vi "VDH-resetCalibrationValues.vi"(11 "VDH-VNA_data_handler in":refnum<class "VDH-VNA_data_handler.lvclass">) -> (3 "VDH-VNA_data_handler out":refnum<class "VDH-VNA_data_handler.lvclass">)   [LabVIEW 2020, in "VDH-VNA_data_handler.lvlib" / "VDH-VNA_data_handler.lvclass"]
uses:
  VDH-VNA_data_handler.lvclass
  VDH-Calibration_info.ctl
  VDH-Calibration_enum.ctl
  VDH-Calibration_factor.ctl
  VDH-calibration_status.ctl
  VDH-SOLT_calib_Status.ctl
  VDH-Calibration_prosess.ctl
  VDH-Calibration_temp_storage.ctl
  VDH-VNA_data_handler.lvclass/VDH-VNA_data_handler.ctl
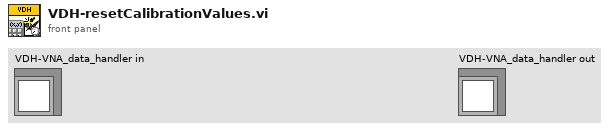
[diagram p1: front panel]
types:
  T1 = typedef "VDH-VNA_data_handler.lvlib/VDH-VNA_data_handler.lvclass/VDH-Calibration_temp_storage.ctl" = cluster{"S11":cdb[][], "Frequency":u64[]}
  T2 = typedef "VDH-VNA_data_handler.lvlib/VDH-VNA_data_handler.lvclass/VDH-calibration_status.ctl" = cluster{"Calib Status":T3, "Calibrated?":bool, "Permativity?":bool, "Progress":T4}
  T3 = typedef "VDH-VNA_data_handler.lvlib/VDH-VNA_data_handler.lvclass/VDH-SOLT_calib_Status.ctl" = cluster{"Short":bool, "Open":bool, "Load":bool, "Through":bool}
  T4 = typedef "VDH-VNA_data_handler.lvlib/VDH-VNA_data_handler.lvclass/VDH-Calibration_prosess.ctl" = cluster{"Progress":bool, "current":T5, "samples to get":u8}
  T5 = typedef "VDH-VNA_data_handler.lvlib/VDH-VNA_data_handler.lvclass/VDH-Calibration_enum.ctl" = enum16{"Non", "Short", "Open", "Load", "Through", "Permativity"}
  T6 = typedef "VDH-VNA_data_handler.lvlib/VDH-VNA_data_handler.lvclass/VDH-Calibration_factor.ctl" = cluster{"A":cdb[], "B":cdb[], "C":cdb[]}
  T7 = typedef "VDH-VNA_data_handler.lvlib/VDH-VNA_data_handler.lvclass/VDH-Calibration_info.ctl" = cluster{"map":map{T5, cdb[]}, "Frequency":u64[]}
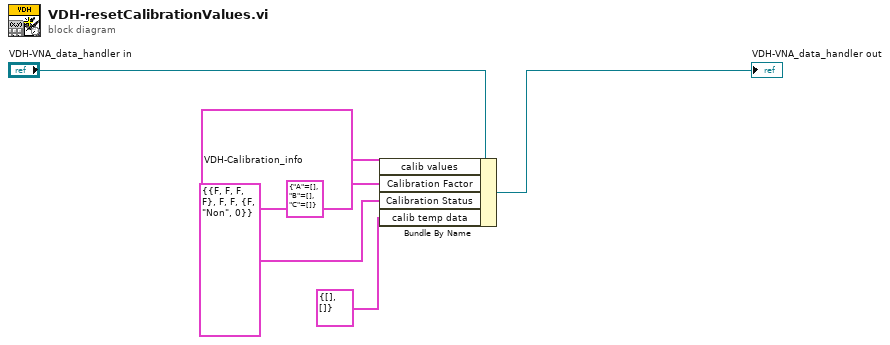
[diagram p0: block diagram]
diagram:
  n1 = Bundle By Name(cluster="VDH-VNA_data_handler in", "calib values"=T7 {"map"={}, "Frequency"=[]} ("SOLT values"), "Calibration Factor"=T6 {"A"=[], "B"=[], "C"=[]}, "Calibration Status"=T2 {"Calib Status"={"Short"=FALSE, "Open"=FALSE, "Load"=FALSE, "Through"=FALSE}, "Calibrated?"=FALSE, "Permativity?"=FALSE, "Progress"={"Progress"=FALSE, "current"=enum."Non", "samples to get"=0}}, "calib temp data"=T1 {"S11"=[], "Frequency"=[]}) -> (→"VDH-VNA_data_handler out":refnum<class "VDH-VNA_data_handler.lvclass">)
